vi "ta_calc_diff.vi"(0 "data in":dbl[][](array[numeric]), 9 "ref in":dbl[][](array[numeric]), 12 "PD values in":dbl[][](array[numeric])) -> (1 "pumped std":dbl[](array[numeric]), 3 "unpumped std":dbl[](array[numeric]), 4 "pumped":dbl[](array[numeric]), 6 "unpumped":dbl[](array[numeric]), 8 "diff std":dbl[](array[numeric]), 10 "diff":dbl[](array[numeric]), 14 "ref std":dbl[](array[numeric]), 15 "ref mean":dbl[](array[numeric]))   [LabVIEW 2019]
uses:
  <vilib>/Analysis/baseanly.llb/Mean (DBL).vi
  <vilib>/Analysis/NI_AALBase.lvlib
panel:
  out "size data":i32[](array[numeric])
  out "size ref":i32[](array[numeric])
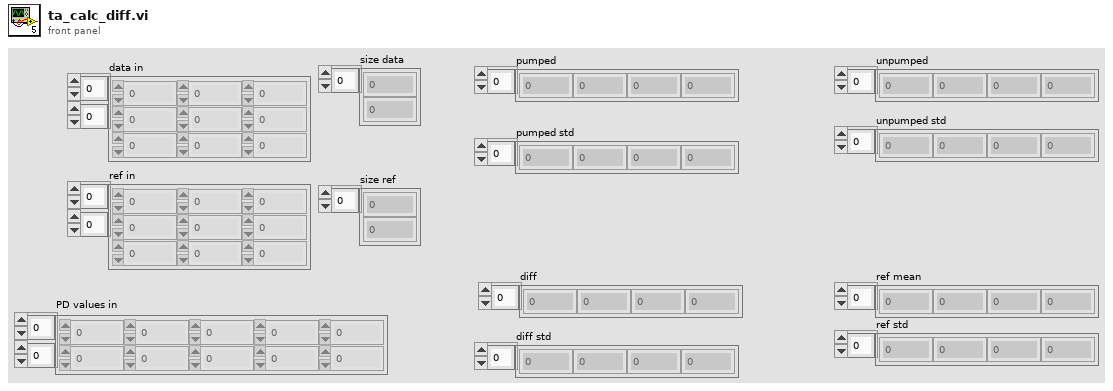
[diagram p1: front panel]
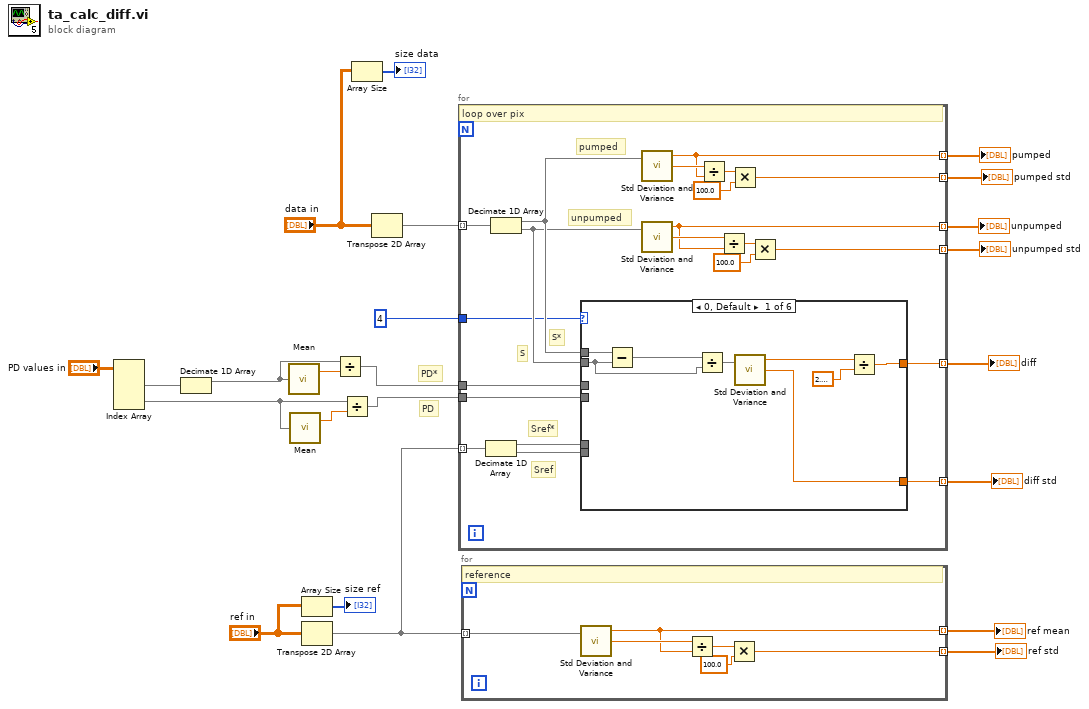
[diagram p0: block diagram]
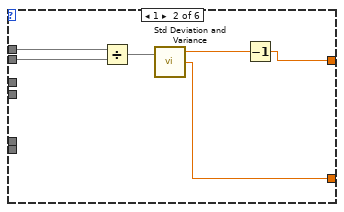
[diagram p2: hidden frame]
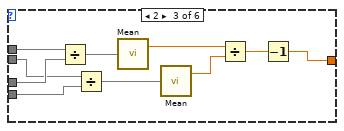
[diagram p3: hidden frame]
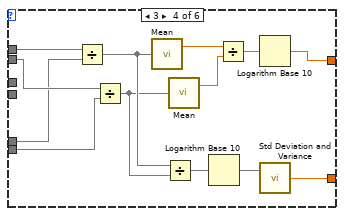
[diagram p4: hidden frame]
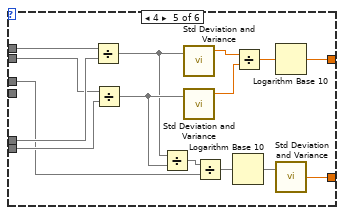
[diagram p5: hidden frame]
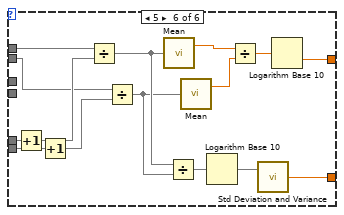
[diagram p6: hidden frame]
diagram:
  # "PD"
  # "PD*"
  n1 = Index Array(array="PD values in") -> (element #1=w4:dbl[], element #2=w7:dbl[])  [unwired: 4 in]
  n2 = Decimate 1D Array(w4) -> (w3:dbl[])  [unwired: 1 out]
  n3 = call-poly <vilib>:"Mean.vi"("X"=w3) -> ("mean"=w8:dbl)  [unwired: 1 out]
  n4 = call-poly <vilib>:"Mean.vi"("X"=w7) -> ("mean"=w6:dbl)  [unwired: 1 out]
  n5 = Array Size(array="ref in") -> (size(s)=→"size ref":i32[])
  n6 = Transpose 2D Array(2D array="ref in") -> (transposed array=w11:dbl[][])
  n7 = Divide(x=w3, y=w8) -> (x/y=w9:dbl[])
  n8 = Divide(x=w7, y=w6) -> (x/y=w5:dbl[])
  n9 = Array Size(array="data in") -> (size(s)=→"size data":i32[])
  n10 = Transpose 2D Array(2D array="data in") -> (transposed array=w17:dbl[][])
  n11 = for {
    tunnel: w17 -> [w42] mode=indexing
    tunnel: [w33] -> w23 mode=indexing
    tunnel: [w40] -> w22 mode=indexing
    tunnel: [w37] -> w15 mode=indexing
    tunnel: [w32] -> w14 mode=indexing
    tunnel: [w31] -> w12 mode=indexing
    tunnel: w9 -> [w26]
    tunnel: w5 -> [w30]
    tunnel: w11 -> [w29] mode=indexing
    tunnel: [w25] -> w2 mode=indexing
    tunnel: 4 -> [w24]
    # "Sref"
    # "Sref*"
    # "S"
    # "S*"
    # "unpumped"
    # "pumped"
    # "loop over pix"
    n12 = Decimate 1D Array(w29) -> (w28:dbl[], w27:dbl[])
    n13 = Decimate 1D Array(w42) -> (w44:dbl[], w43:dbl[])
    n14 = case shown="0, Default" w24 {
      tunnel: w44 -> [w52 w58 w68 w81 w94 w105]
      tunnel: w43 -> [w51 w57 w66 w80 w92 w104]
      tunnel: [w49 w56 w59 w75 w95 w106] -> w31
      tunnel: w26 -> [_ _ w67 _ w83 _]
      tunnel: w30 -> [_ _ w65 _ _ _]
      tunnel: w28 -> [_ _ _ w74 w93 w103]
      tunnel: w27 -> [_ _ _ w79 w91 w102]
      tunnel: [w47 w53 _ w69 w86 w97] -> w25
      frame 0, Default {
        n15 = Subtract(x=w52, y=w51) -> (x-y=w45:dbl[])
        n16 = Divide(x=w45, y=w51) -> (x/y=w46:dbl[])
        n17 = call <vilib>:"Std Deviation and Variance.vi"("X"=w46) -> ("mean"=w48:dbl, "standard deviation"=w47:dbl)  [unwired: 1 in, 1 out]
        n18 = Divide(x=w48, y=2.302585092994046) -> (x/y=w49:dbl)
      }
      frame 1 {
        n19 = Divide(x=w58, y=w57) -> (x/y=w55:dbl[])
        n20 = call <vilib>:"Std Deviation and Variance.vi"("X"=w55) -> ("mean"=w54:dbl, "standard deviation"=w53:dbl)  [unwired: 1 in, 1 out]
        n21 = Decrement(x=w54) -> (x-1=w56:dbl)
      }
      frame 2 {
        n22 = Divide(x=w68, y=w67) -> (x/y=w64:dbl[])
        n23 = Divide(x=w66, y=w65) -> (x/y=w63:dbl[])
        n24 = call-poly <vilib>:"Mean.vi"("X"=w64) -> ("mean"=w62:dbl)  [unwired: 1 out]
        n25 = call-poly <vilib>:"Mean.vi"("X"=w63) -> ("mean"=w61:dbl)  [unwired: 1 out]
        n26 = Divide(x=w62, y=w61) -> (x/y=w60:dbl)
        n27 = Decrement(x=w60) -> (x-1=w59:dbl)
      }
      frame 3 {
        n28 = Divide(x=w81, y=w74) -> (x/y=w73:dbl[])
        n29 = Divide(x=w80, y=w79) -> (x/y=w72:dbl[])
        n30 = call-poly <vilib>:"Mean.vi"("X"=w73) -> ("mean"=w78:dbl)  [unwired: 1 out]
        n31 = Divide(x=w73, y=w72) -> (x/y=w71:dbl[])
        n32 = call-poly <vilib>:"Mean.vi"("X"=w72) -> ("mean"=w77:dbl)  [unwired: 1 out]
        n33 = Logarithm Base 10(1:w71) -> (0:w70:dbl[])
        n34 = Divide(x=w78, y=w77) -> (x/y=w76:dbl)
        n35 = Logarithm Base 10(1:w76) -> (0:w75:dbl)
        n36 = call <vilib>:"Std Deviation and Variance.vi"("X"=w70) -> ("standard deviation"=w69:dbl)  [unwired: 1 in, 2 out]
      }
      frame 4 {
        n37 = Divide(x=w94, y=w93) -> (x/y=w85:dbl[])
        n38 = Divide(x=w92, y=w91) -> (x/y=w88:dbl[])
        n39 = Divide(x=w85, y=w88) -> (x/y=w84:dbl[])
        n40 = call <vilib>:"Std Deviation and Variance.vi"("X"=w85) -> ("mean"=w90:dbl)  [unwired: 1 in, 2 out]
        n41 = call <vilib>:"Std Deviation and Variance.vi"("X"=w88) -> ("mean"=w89:dbl)  [unwired: 1 in, 2 out]
        n42 = Divide(x=w84, y=w83) -> (x/y=w82:dbl[])
        n43 = Logarithm Base 10(1:w82) -> (0:w87:dbl[])
        n44 = Divide(x=w90, y=w89) -> (x/y=w96:dbl)
        n45 = Logarithm Base 10(1:w96) -> (0:w95:dbl)
        n46 = call <vilib>:"Std Deviation and Variance.vi"("X"=w87) -> ("standard deviation"=w86:dbl)  [unwired: 1 in, 2 out]
      }
      frame 5 {
        n47 = Increment(x=w103) -> (x+1=w110:dbl[])
        n48 = Increment(x=w102) -> (x+1=w111:dbl[])
        n49 = Divide(x=w105, y=w110) -> (x/y=w101:dbl[])
        n50 = Divide(x=w104, y=w111) -> (x/y=w100:dbl[])
        n51 = call-poly <vilib>:"Mean.vi"("X"=w101) -> ("mean"=w107:dbl)  [unwired: 1 out]
        n52 = Divide(x=w101, y=w100) -> (x/y=w99:dbl[])
        n53 = call-poly <vilib>:"Mean.vi"("X"=w100) -> ("mean"=w108:dbl)  [unwired: 1 out]
        n54 = Logarithm Base 10(1:w99) -> (0:w98:dbl[])
        n55 = Divide(x=w107, y=w108) -> (x/y=w109:dbl)
        n56 = call <vilib>:"Std Deviation and Variance.vi"("X"=w98) -> ("standard deviation"=w97:dbl)  [unwired: 1 in, 2 out]
        n57 = Logarithm Base 10(1:w109) -> (0:w106:dbl)
      }
    }
    n58 = call <vilib>:"Std Deviation and Variance.vi"("X"=w44) -> ("mean"=w40:dbl, "standard deviation"=w41:dbl)  [unwired: 1 in, 1 out]
    n59 = call <vilib>:"Std Deviation and Variance.vi"("X"=w43) -> ("mean"=w33:dbl, "standard deviation"=w34:dbl)  [unwired: 1 in, 1 out]
    n60 = Divide(x=w41, y=w40) -> (x/y=w39:dbl)
    n61 = Divide(x=w34, y=w33) -> (x/y=w36:dbl)
    n62 = Multiply(x=w39, y=100.0) -> (x*y=w37:dbl)
    n63 = Multiply(x=w36, y=100.0) -> (x*y=w32:dbl)
  }
  "diff" <- w12
  "unpumped" <- w23
  "pumped" <- w22
  "pumped std" <- w15
  "unpumped std" <- w14
  "diff std" <- w2
  n64 = for {
    tunnel: w11 -> [w117] mode=indexing
    tunnel: [w115] -> w21 mode=indexing
    tunnel: [w112] -> w16 mode=indexing
    # "reference"
    n65 = call <vilib>:"Std Deviation and Variance.vi"("X"=w117) -> ("mean"=w115:dbl, "standard deviation"=w116:dbl)  [unwired: 1 in, 1 out]
    n66 = Divide(x=w116, y=w115) -> (x/y=w114:dbl)
    n67 = Multiply(x=w114, y=100.0) -> (x*y=w112:dbl)
  }
  "ref mean" <- w21
  "ref std" <- w16
